vi "Convert Source VI to Resource Data.vi"(8 "error in (no error)":errorcluster, 10 "Use VTT?":bool, 11 "Source VI Ref":refnum<vi>) -> (0 "error out":errorcluster, 1 "BD Resource Data":string, 2 "FP Resource Data":string, 3 "Resources":T1[](array[typedef]))   [LabVIEW 2026, in "VILab.lvlib"]
uses:
  VILab.lvlib
  CTLs/Resource.ctl
  Find Resource by Type (String).vi
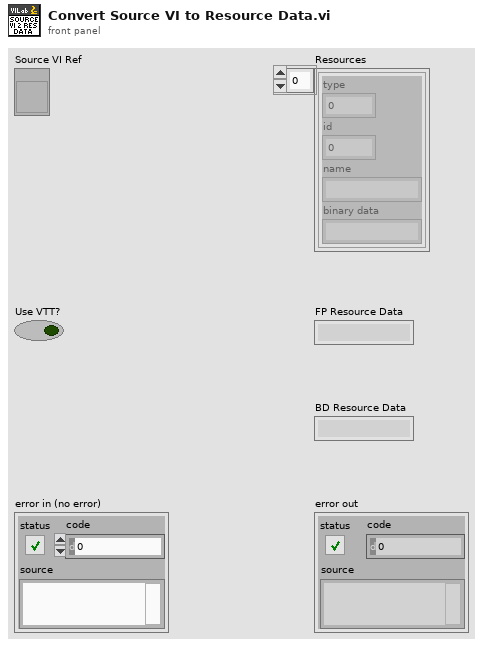
[diagram p1: front panel]
types:
  T1 = typedef "VILab.lvlib/Resource.ctl" = cluster{"type":u32, "id":i32, "name":string, "binary data":string}
  T2 = typedef "VILab.lvlib/Heap Save Format.ctl" = u16
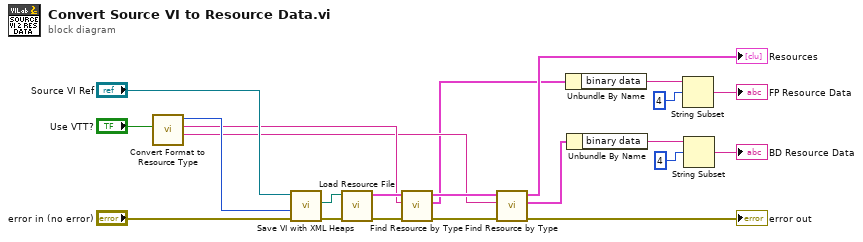
[diagram p0: block diagram]
diagram:
  n1 = call "Convert Format to Resource Type.vi"("Use VTT?"="Use VTT?") -> ("BD Resource Type"=w6:string, "FP Resource Type"=w7:string, "Heap Save Format"=w13:T2)  [unwired: 8 in]
  n2 = call "Save VI with XML Heaps.vi"("error in (no error)"="error in (no error)", "Heap Save Format (1=XML)"=w13, "VI Refnum In"="Source VI Ref") -> ("error out"=w16:errorcluster, "VI Path out"=w21:path)  [unwired: 6 in, 1 out]
  n3 = call "Load Resource File.vi"("error in (no error)"=w16, "Resource File"=w21) -> ("error out"=w12:errorcluster, "Resources"=w8:T1[])  [unwired: 7 in, 1 out]
  n4 = call-poly "Find Resource by Type.vi"("error in (no error)"=w12, "Resource Type"=w7, "Resources"=w8) -> ("error out"=w11:errorcluster, "Resource"=w2:T1, "Resources out"=w22:T1[])  [unwired: 4 in, 2 out]
  n5 = call-poly "Find Resource by Type.vi"("error in (no error)"=w11, "Resource Type"=w6, "Resources"=w22) -> ("error out"=→"error out":errorcluster, "Resource"=w1:T1, "Resources out"=→"Resources":T1[])  [unwired: 4 in, 2 out]
  n6 = Unbundle By Name(w2) -> ("binary data"=w20:string)
  n7 = Unbundle By Name(w1) -> ("binary data"=w17:string)
  n8 = String Subset(string=w20, offset (0)=4) -> (substring=→"FP Resource Data":string)  [unwired: 1 in]
  n9 = String Subset(string=w17, offset (0)=4) -> (substring=→"BD Resource Data":string)  [unwired: 1 in]
